vi "Retrieve Token String.vi"(2 "Offset (0)":i32, 3 "input string":string) -> (0 "token string":string, 1 "output string":string)   [LabVIEW 2010]
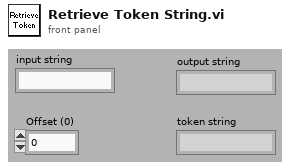
[diagram p1: front panel]
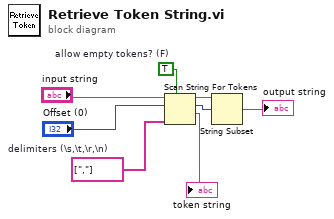
[diagram p0: block diagram]
diagram:
  w1 = TRUE  # allow empty tokens? (F)
  w2 = string[] [","]  # delimiters (\s,\t,\r,\n)
  n1 = Scan String For Tokens(5:w1, 6:w2, 8:"Offset (0)", 9:"input string") -> (1:→"token string":string, 2:w7:i32, 3:w6:string)  [unwired: 2 in, 1 out]
  n2 = String Subset(string=w6, offset (0)=w7) -> (substring=→"output string":string)  [unwired: 1 in]
